vi "Create Packet Collection.vi"(10 "Packets":refnum<class "ControlPacket.lvclass">[](array[class])) -> (3 "PacketCollection":refnum<class "PacketCollection.lvclass">)   [LabVIEW 2013, in "MQTT Server.lvlib" / "PacketCollection.lvclass"]
uses:
  PacketCollection.lvclass
  <vilib>/LabVIEW Open Source Project/MQTT Control Packets/Control Packets/ControlPacket/ControlPacket.lvclass
  PacketCollection.lvclass/PacketCollection.ctl
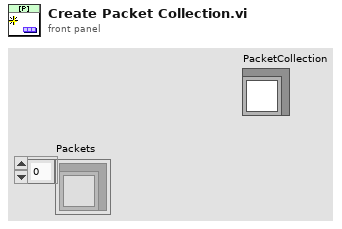
[diagram p1: front panel]
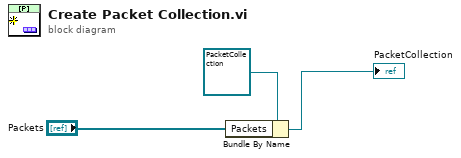
[diagram p0: block diagram]
diagram:
  n1 = Bundle By Name(cluster=refnum<class "PacketCollection.lvclass"> refnum ("PacketCollection in"), "Packets"="Packets") -> (→"PacketCollection":refnum<class "PacketCollection.lvclass">)
